vi "Propagate Error.vi"(8 "error in (no error)":errorcluster, 11 "Process in":refnum<class "Process.lvclass">) -> (0 "error out":errorcluster, 3 "Process out":refnum<class "Process.lvclass">)   [LabVIEW 2021, in "Process.lvlib" / "Process.lvclass"]
uses:
  Process.lvclass
  Process.lvclass/Process.ctl
  AAM/AAM/LVCAM/LVCAM.lvclass
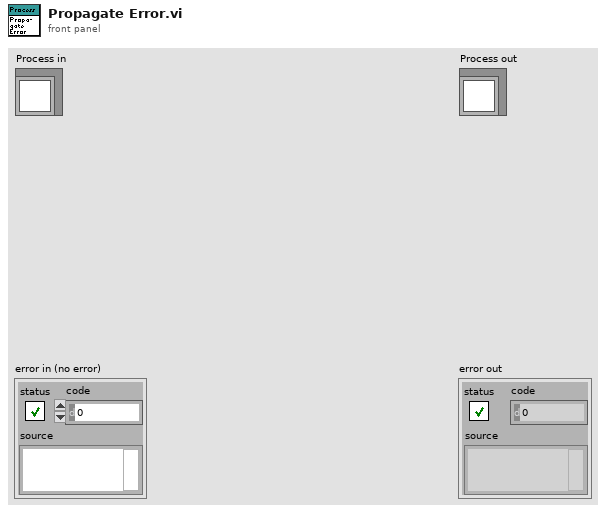
[diagram p1: front panel]
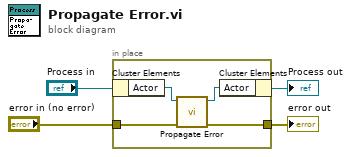
[diagram p0: block diagram]
diagram:
  n1 = in-place {
    in-place-border: "error in (no error)" -> [w6]
    in-place-border: [w5] -> w1
    n2 = in-place-cluster #1("Process in") -> ("Actor"=w8:refnum<class "LVCAM.lvclass">)
    n3 = call-dynamic "Propagate Error.vi"("error in (no error)"=w6, "Propagate Error in"=w8) -> ("error out"=w5:errorcluster, "Propagate Error out"=w7:refnum<class "LVCAM.lvclass">)  [unwired: 8 in]
    n4 = in-place-cluster #1("Actor"=w7) -> (→"Process out":refnum<class "Process.lvclass">)
  }
  "error out" <- w1
